vi "LJM_eWriteNames.vi"(0 "Handle In":i32, 1 "NumFrames":i32, 5 "aNames":string[](array[string]), 9 "aValuesIn":dbl[](array[numeric]) format="%.2f", 11 "error in":errorcluster) -> (4 "Handle Out":i32, 14 "ErrorAddress":i32, 15 "error out":errorcluster)   [LabVIEW 2017]
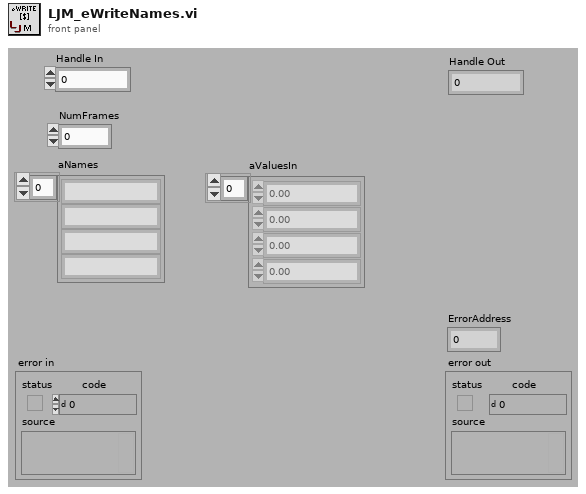
[diagram p1: front panel]
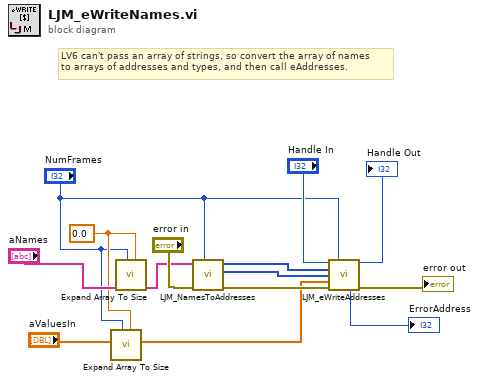
[diagram p0: block diagram]
diagram:
  w12 = 0.0 ("Default Value")
  # "LV6 can't pass an array of strings, so convert the array of names\nto arrays of addresses and types, and then call eAddresses."
  n1 = call <userlib>:"Expand Array To Size.vi"("Default Value"=w12, "# Elements"="NumFrames", "DBL Array In"="aValuesIn") -> ("DBL Array Out"=w1:dbl[])  [unwired: 4 in, 4 out]
  n2 = call <userlib>:"Expand Array To Size.vi"("Default Value"=w12, "# Elements"="NumFrames", "String Array In"="aNames") -> ("String Array Out"=w10:string[])  [unwired: 4 in, 4 out]
  n3 = call <userlib>:"LJM_NamesToAddresses.vi"("NumFrames (Auto-Detect)"="NumFrames", "error in"="error in", "aNames"=w10) -> ("error out"=w9:errorcluster, "aTypes"=w2:i32[], "aAddresses"=w3:i32[])  [unwired: 6 in]
  n4 = call "LJM_eWriteAddresses.vi"("Handle In"="Handle In", "NumFrames"="NumFrames", "aAddresses"=w3, "aTypes"=w2, "aValues"=w1, "error in"=w9) -> ("Handle Out"=→"Handle Out":i32, "ErrorAddress"=→"ErrorAddress":i32, "error out"=→"error out":errorcluster)  [unwired: 7 in]
